vi "OpenLoop_SaveExp.vi"() -> ()   [LabVIEW 2014]
uses:
  <vilib>/Platform/TimedLoop/XDataNode/timing_clust.ctl
  <vilib>/Platform/TimedLoop/XDataNode/nitl_modes.ctl
  <vilib>/Platform/TimedLoop/XDataNode/wakeup.ctl
  <vilib>/myRIO/Instrument Drivers/Onboard IO/AI/typedefs/AI Reference.ctl
  <vilib>/myRIO/Common/Instrument Driver Framework/Utilities/typedefs/myRIO Generic Hardware Reference.ctl
  <vilib>/myRIO/Common/Instrument Driver Framework/Utilities/typedefs/Hardware Version Enum.ctl
  <vilib>/myRIO/Common/Instrument Driver Framework/Utilities/typedefs/myRIO v1.0 Reference.ctl
  <vilib>/myRIO/Common/Instrument Driver Framework/Utilities/typedefs/Generic FPGA Reference.ctl
  <vilib>/myRIO/Common/Instrument Driver Framework/myRIO v1.0/AI/typedefs/AI Channels List.ctl
  <vilib>/myRIO/Common/Instrument Driver Framework/myRIO v1.0/AI/typedefs/AI Channels Enum.ctl
  <vilib>/myRIO/Common/Instrument Driver Framework/Utilities/typedefs/Analog Scaling Constants List.ctl
  <vilib>/myRIO/Common/Instrument Driver Framework/Utilities/typedefs/Analog Scaling Constants.ctl
  <vilib>/userdefined/High Color/nirio_resource_hc.ctl
  <vilib>/myRIO/Instrument Drivers/Onboard IO/AO/typedefs/AO Reference.ctl
  <vilib>/myRIO/Common/Instrument Driver Framework/myRIO v1.0/AO/typedefs/AO Channels List.ctl
  <vilib>/myRIO/Common/Instrument Driver Framework/myRIO v1.0/AO/typedefs/AO Channels Enum.ctl
  <vilib>/myRIO/Common/Instrument Driver Framework/myRIO v1.0/AI/vis/myRIO v1.1 Open AI.vi
  <vilib>/myRIO/Common/Instrument Driver Framework/myRIO v1.0/AO/vis/myRIO v1.1 Open AO.vi
  <vilib>/myRIO/Common/Instrument Driver Framework/Utilities/vis/Validate Channels.vi
  <vilib>/myRIO/Common/Instrument Driver Framework/myRIO v1.0/AI/vis/myRIO v1.0 Reserve AI.vi
  <vilib>/myRIO/Common/Instrument Driver Framework/myRIO v1.0/AO/vis/myRIO v1.0 Reserve AO.vi
  <vilib>/myRIO/Common/Instrument Driver Framework/myRIO v1.0/UART/vis/myRIO v1.0 Close UART.vi
  <vilib>/myRIO/Common/Instrument Driver Framework/myRIO v1.0/AI/vis/myRIO v1.0 Build MUX Configuration AI.vi
  <vilib>/myRIO/Common/Instrument Driver Framework/myRIO v1.0/Resource Manager/vis/myRIO v1.0 Reserve Channel List.vi
  <vilib>/myRIO/Common/Instrument Driver Framework/myRIO v1.0/AO/vis/myRIO v1.0 Build MUX Configuration AO.vi
  <vilib>/myRIO/Common/Instrument Driver Framework/myRIO v1.0/Resource Manager/vis/myRIO v1.0 Reserve Channel.vi
  <vilib>/myRIO/Common/Instrument Driver Framework/myRIO v1.0/Resource Manager/vis/myRIO v1.0 Unreserve Channel.vi
  <vilib>/myRIO/Common/Instrument Driver Framework/myRIO v1.0/Resource Manager/vis/myRIO v1.0 Build Mutex Name.vi
  <vilib>/Utility/VariantDataType/GetNumericInfo.vi
  <vilib>/Utility/error.llb/Error Cluster From Error Code.vi
  <vilib>/myRIO/Common/Instrument Driver Framework/myRIO v1.0/myRIO v1.1 Open.vi
  <vilib>/myRIO/Common/Instrument Driver Framework/myRIO v1.0/AI/vis/myRIO v1.0 Get Scaling Constants AI.vi
  <vilib>/myRIO/Common/Instrument Driver Framework/Utilities/vis/IO Manager.vi
  <vilib>/myRIO/Common/Instrument Driver Framework/Utilities/vis/Configuration Manager.vi
  <vilib>/myRIO/Common/Instrument Driver Framework/myRIO v1.0/myRIO v1.0 Close.vi
  <vilib>/myRIO/Common/Instrument Driver Framework/myRIO v1.0/AO/vis/myRIO v1.0 Get Scaling Constants AO.vi
  <vilib>/myRIO/Common/Instrument Driver Framework/myRIO v1.0/AI/vis/myRIO v1.0 Read AI.vi
  <vilib>/myRIO/Common/Instrument Driver Framework/myRIO v1.0/AO/vis/myRIO v1.0 Write AO.vi
  <vilib>/myRIO/Common/Instrument Driver Framework/Utilities/vis/FPGA Ref Manager.vi
  <vilib>/myRIO/Common/Instrument Driver Framework/myRIO v1.0/myRIO v1.0 Reset FPGA.vi
  <vilib>/myRIO/Common/Instrument Driver Framework/myRIO v1.0/IRQ/vis/myRIO v1.0 IRQ Info FGV.vi
  <vilib>/myRIO/Common/Instrument Driver Framework/myRIO v1.0/IRQ/vis/myRIO v1.0 Timer IRQ Info FGV.vi
  <vilib>/myRIO/Common/Instrument Driver Framework/myRIO v1.0/IRQ/vis/myRIO v1.0 ISR Agent.vi
  <vilib>/Platform/TimedLoop/XDataNode/XDataNode.xnode
  <vilib>/myRIO/Instrument Drivers/Onboard IO/AI/vis/myRIO AI Open.xnode
  <vilib>/myRIO/Instrument Drivers/Onboard IO/AO/vis/myRIO AO Open.xnode
  <vilib>/myRIO/Instrument Drivers/Utilities/Utilities.lvlib
  <vilib>/Platform/TimedLoop/XDataNode/XDNodeRunTimeDep.lvlib
  <vilib>/myRIO/Instrument Drivers/Onboard IO/AI/AI.lvlib
  <vilib>/myRIO/Instrument Drivers/Onboard IO/AO/AO.lvlib
panel:
  in  "Intensidade do acionamento":sgl(slide) scale=-10.0..10.0
  out "Waveform Chart":dbl[][](graph)
  in  "stop":bool
  out "error out":errorcluster
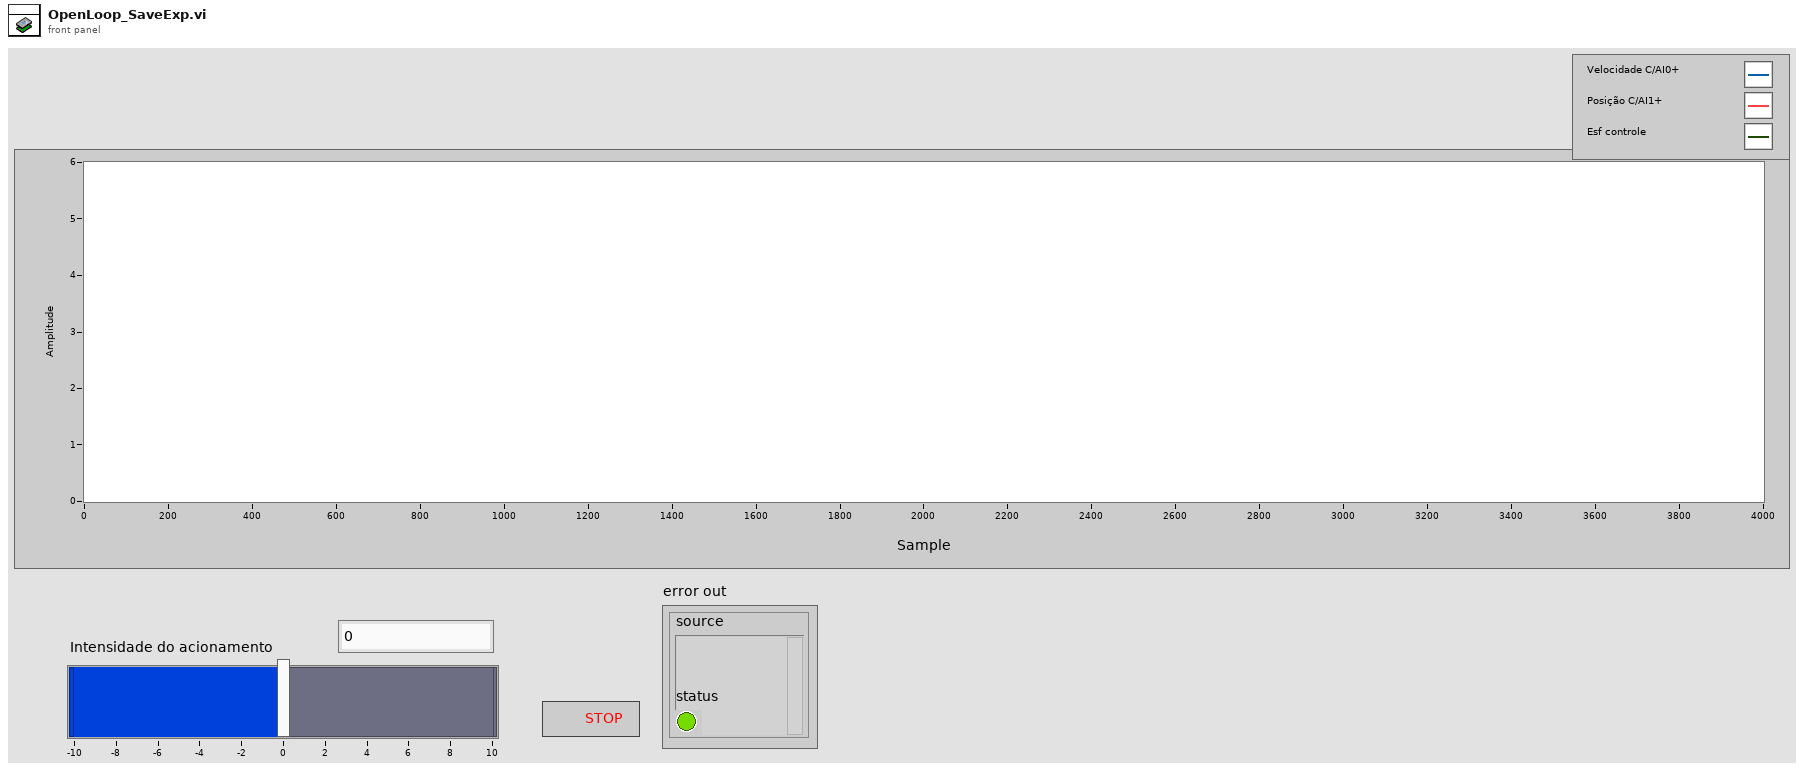
[diagram p1: front panel]
types:
  T1 = typedef "nirio_resource_hc.ctl" = tag
  T2 = typedef "Hardware Version Enum.ctl" = enum16{"Unknown", "myRIO-1900", "myRIO-1950"}
  T3 = typedef "XDNodeRunTimeDep.lvlib/timing_clust.ctl" = cluster{"Expected End [f-1]":u64, "Actual End [f-1]":u64, "Finished Late? [f-1]":bool, "Expected End [i-1]":u64, "Actual End [i-1]":u64, "Finished Late? [i-1]":bool, "Expected Start [i]":u64, "Actual Start [i]":u64, "Expected Start [f]":u64, "Actual Start [f]":u64, "Source Name":string, "Structure Name":string, "Period":i64, "Deadline":i64, "Offset":i64, "Start":i64, "Priority":i32, "Timeout":i32, "Mode":T4, "Wakeup Reason":T5, "Error":errorcluster, "Source Type":string, "Secondary Source Type":string, "Global End Time":u64, "Global Start Time":u64, "Frame Duration":u64, "Iteration Duration":u64, "Assigned CPU":i32, "I/O Scan Engine Mode":u32}
  T4 = typedef "XDNodeRunTimeDep.lvlib/nitl_modes.ctl" = enum32{"No Change", "Process missed periods, maintain original phase", "Discard missed periods, maintain original phase", "Process missed periods, ignore original phase", "Discard missed periods, ignore original phase"}
  T5 = typedef "XDNodeRunTimeDep.lvlib/wakeup.ctl" = enum32{"Normal", "Aborted", "Asynchronous wakeup", "Timing source error", "Timed loop error", "Timeout"}
  T6 = enum16{"open", "replace", "create", "open or create", "replace or create", "replace or create with confirmation"}
  T7 = typedef "AI.lvlib/AI Reference.ctl" = cluster{"myRIO Reference":T8, "AI Channels List":T11, "AI Scaling Constants List":T13}
  T8 = typedef "myRIO Generic Hardware Reference.ctl" = cluster{"myRIO Model":T2, "myRIO Hardware Reference":T9}
  T9 = typedef "myRIO v1.0 Reference.ctl" = cluster{"Generic FPGA Reference":T10, "Allow multiple opens":bool}
  T10 = typedef "Generic FPGA Reference.ctl" = refnum<k20>
  T11 = typedef "AI Channels List.ctl" = T12[]
  T12 = typedef "AI Channels Enum.ctl" = enum16{"Not Connected", "AudioIn/Left", "AudioIn/Right", "C/AI0", "C/AI1", "A/AI0", "A/AI1", "A/AI2", "A/AI3", "B/AI0", "B/AI1", "B/AI2", "B/AI3"}
  T13 = typedef "Analog Scaling Constants List.ctl" = T14[]
  T14 = typedef "Analog Scaling Constants.ctl" = cluster{"LSB Weight (Volts)":dbl, "Offset (Volts)":dbl, "Signed?":bool}
  T15 = typedef "AO.lvlib/AO Reference.ctl" = cluster{"myRIO Reference":T8, "AO Channel List":T16, "AO Scaling Constant List":T13}
  T16 = typedef "AO Channels List.ctl" = T17[]
  T17 = typedef "AO Channels Enum.ctl" = enum16{"Not Connected", "AudioOut/Left", "AudioOut/Right", "C/AO0", "C/AO1", "A/AO0", "A/AO1", "B/AO0", "B/AO1"}
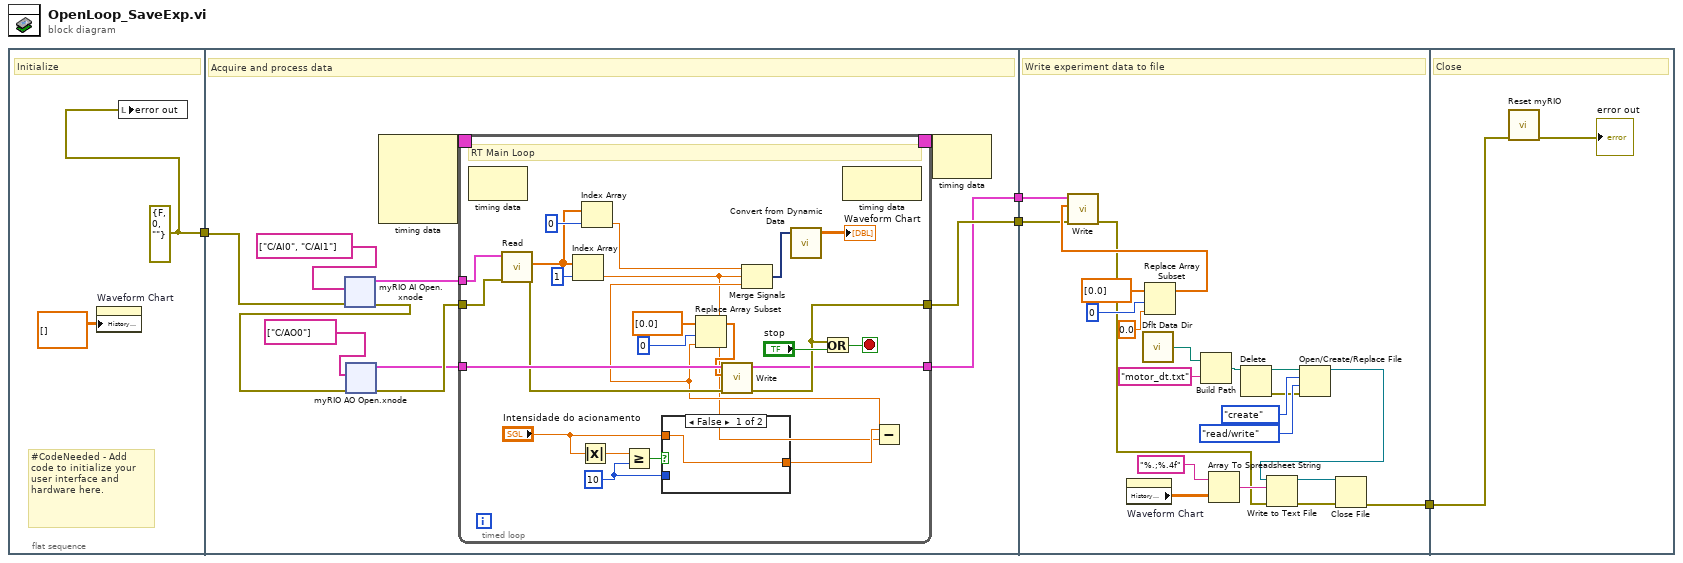
[diagram p0: block diagram]
diagram:
  n1 = flat-sequence {
    tunnel: [w5] -> w4
    tunnel: w4 -> [w15]
    tunnel: [w13] -> w3
    tunnel: [w7] -> w2
    tunnel: w3 -> [w98]
    tunnel: w2 -> [w97]
    tunnel: [w89] -> w1
    tunnel: w1 -> [w105]
    frame #0 {
      w5 = errorcluster {"status"=FALSE, "code"=0, "source"=""} ("error out")
      # "#CodeNeeded - Add code to initialize your user interface and hardware here."
      # "Initialize"
      n2 = property on="Waveform Chart" class="WFChart (strict)"("History Data"=dbl[][] []) -> ()  [unwired: 2 in, 2 out]
      n3 = local write "error out"(w5) -> ()
    }
    frame #1 {
      # "Acquire and process data"
      n4 = xnode "myRIO AI Open.xnode"("error in (no error)"=w15, "Channel Names"=tag[] ["C/AI0", "C/AI1"]) -> ("error out"=w9:errorcluster, "AI Ref Out"=w14:T7)  [unwired: 1 in]
      n5 = xnode "myRIO AO Open.xnode"("error in (no error)"=w9, "Channel Names"=tag[] ["C/AO0"]) -> ("error out"=w10:errorcluster, "AO Ref Out"=w8:T15)  [unwired: 1 in]
      n6 = node-c288() -> (w17:T3)  [unwired: 4 in]
      n7 = timed-loop {
        timing: w17 -> [_]
        timing-out: [_] -> w16
        tunnel: w14 -> [w75]
        tunnel: w10 -> [w74]
        tunnel: [w68] -> w13
        tunnel: w8 -> [w70]
        tunnel: [w60] -> w7
        stop <- w76 stop-if-true
        w61 = 10
        # "RT Main Loop"
        n8 = node-c288() -> ()  [unwired: 1 in, 1 out]
        n9 = call <vilib>:"Read.vi"("error in (no error)"=w74, "AI Ref In"=w75) -> ("error out"=w69:errorcluster, "Values"=w71:dbl[])  [unwired: 7 in, 1 out]
        n10 = Index Array(array=w71, index=1) -> (element=w54:dbl)
        n11 = Absolute Value(x="Intensidade do acionamento") -> (abs(x)=w63:sgl)
        n12 = Index Array(array=w71, index=0) -> (element=w59:dbl)
        n13 = Greater Or Equal?(x=w63, y=w61) -> (x >= y?=w64:bool)
        n14 = case shown="False" w64 {
          tunnel: [w78 w79] -> w56
          tunnel: "Intensidade do acionamento" -> [w78 _]
          tunnel: w61 -> [_ w79]
          frame False {
          }
          frame True {
          }
        }
        n15 = node-c288() -> ()  [unwired: 1 in, 1 out]
        n16 = Subtract(x=w56, y=w54) -> (x-y=w55:dbl)
        n17 = Replace Array Subset(array=dbl[] [0.0] ("Values"), new element=w55, index=0) -> (w67:dbl[])
        n18 = call <vilib>:"Write.vi"("error in (no error)"=w69, "Values"=w67, "AO Ref In"=w70) -> ("error out"=w68:errorcluster, "AO Ref Out"=w60:T15)  [unwired: 6 in]
        n19 = Merge Signals(w59, w54, w55) -> (w58:dynamicdata)
        n20 = call "Convert from Dynamic Data"("Dynamic Data Type"=w58) -> ("Array"=→"Waveform Chart":dbl[][])  [unwired: 3 in]
        n21 = Or(x=w68, y="stop") -> (x .or. y?=w76:bool)
      }
      n22 = node-c288(w16) -> ()  [unwired: 1 out]
    }
    frame #2 {
      # "Write experiment data to file"
      n23 = property on="Waveform Chart" class="WFChart (strict)"() -> ("History Data"=w86:dbl[][])  [unwired: 2 in, 2 out]
      n24 = call <vilib>:"Dflt Data Dir.vi"() -> ("App:Default Data Directory"=w85:path)
      n25 = Replace Array Subset(array=dbl[] [0.0] ("Values"), new element=0.0 ("new element/subarray"), index=0) -> (w99:dbl[])
      n26 = call <vilib>:"Write.vi"("error in (no error)"=w98, "Values"=w99, "AO Ref In"=w97) -> ("error out"=w84:errorcluster)  [unwired: 6 in, 1 out]
      n27 = Build Path(base path=w85, name or relative path="motor_dt.txt") -> (appended path=w94:path)
      n28 = Array To Spreadsheet String(array=w86, 3:"%.;%.4f" ("format string")) -> (spreadsheet string=w103:string)  [unwired: 1 in]
      n29 = Delete(path (use dialog)=w94) -> (deleted path=w93:path, error out=w88:errorcluster)  [unwired: 4 in, 1 out]
      n30 = Open/Create/Replace File(file path (use dialog)=w93, error in=w88, operation (0:open)=T6."create", access (0:read/write)=enum16{"read/write", "read-only", "write-only"}."read/write") -> (refnum out=w92:refnum<file>)  [unwired: 4 out]
      n31 = Write to Text File(file (use dialog)=w92, text=w103, error in=w84) -> (refnum out=w90:refnum<file>, error out=w91:errorcluster)  [unwired: 1 in, 1 out]
      n32 = Close File(refnum=w90, error in=w91) -> (error out=w89:errorcluster)  [unwired: 1 out]
    }
    frame #3 {
      # "Close"
      n33 = call <vilib>:"Reset myRIO.vi"("error in (no error)"=w105) -> ("error out"=→"error out":errorcluster)  [unwired: 10 in]
    }
  }
